vi "Read.vi"(11 "ReplyValue in":refnum<class "ReplyValue.lvclass">) -> (2 "TcpPayload":T1)   [LabVIEW 2020, in "Vecto.lvlib" / "ReplyValue.lvclass"]
uses:
  ReplyValue.lvclass
  proto/TcpPayload/Data.ctl
  ReplyValue.lvclass/ReplyValue.ctl
  proto/TcpPayload/TcpPayload.lvlib
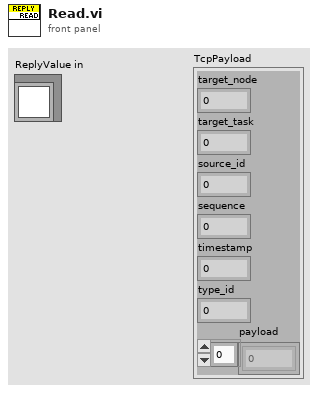
[diagram p1: front panel]
types:
  T1 = typedef "TcpPayload.lvlib/Data.ctl" = cluster{"target_node":u32, "target_task":u32, "source_id":u32, "sequence":u32, "timestamp":u64, "type_id":u32, "payload":u8[]}
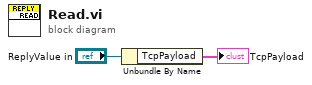
[diagram p0: block diagram]
diagram:
  n1 = Unbundle By Name("ReplyValue in") -> ("TcpPayload"=→"TcpPayload":T1)
